vi "HelloWorld.vi"() -> ()   [LabVIEW 2018]
panel:
  out "String":string
  in  "Numeric 4":dbl
  in  "New Sidebar 2":dbl(slide) scale=0.0..10.0
  out "Numeric 3":dbl
  out "Tank 2":dbl(slide) scale=0.0..100.0
  in  "stop 2":bool
  out "loop info 2":dbl
  out "loop info":dbl
  in  "stop":bool
  out "Tank":dbl(slide) scale=0.0..100.0
  out "Numeric 2":dbl
  in  "New Sidebar":dbl(slide) scale=0.0..10.0
  in  "Numeric":dbl
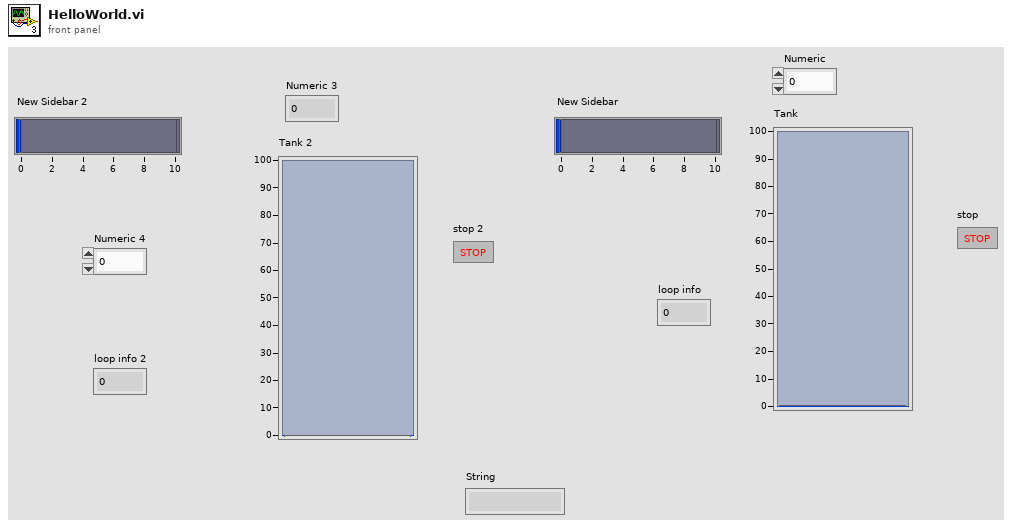
[diagram p1: front panel]
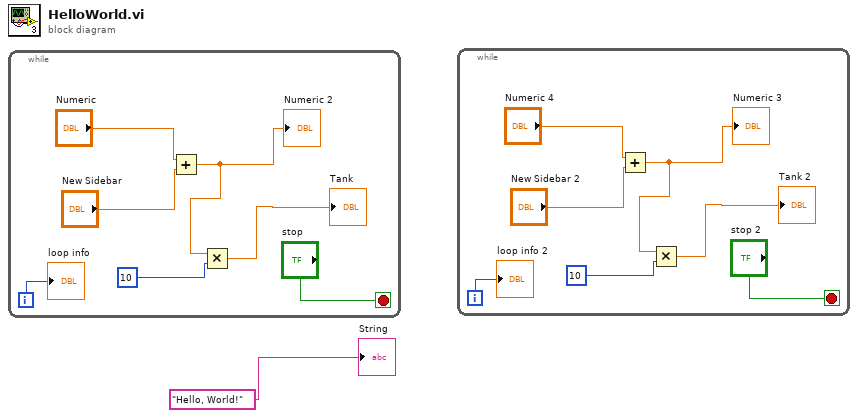
[diagram p0: block diagram]
diagram:
  n1 = while {
    i -> [w2]
    stop <- "stop" stop-if-true
    n2 = Add(x="Numeric", y="New Sidebar") -> (x+y=w4:dbl)
    "Numeric 2" <- w4
    n3 = Multiply(x=w4, y=10) -> (x*y=→"Tank":dbl)
    "loop info" <- w2
  }
  n4 = while {
    i -> [w9]
    stop <- "stop 2" stop-if-true
    n5 = Add(x="Numeric 4", y="New Sidebar 2") -> (x+y=w11:dbl)
    "Numeric 3" <- w11
    n6 = Multiply(x=w11, y=10) -> (x*y=→"Tank 2":dbl)
    "loop info 2" <- w9
  }
  "String" <- "Hello, World!"
